vi "How to Calculate and Display Roots.vi"() -> ()   [LabVIEW 2020]
panel:
  out "Less Than 0":bool
  out "Greater than 0":bool
  out "D":dbl
  in  "C":dbl
  in  "B":dbl
  in  "A":dbl
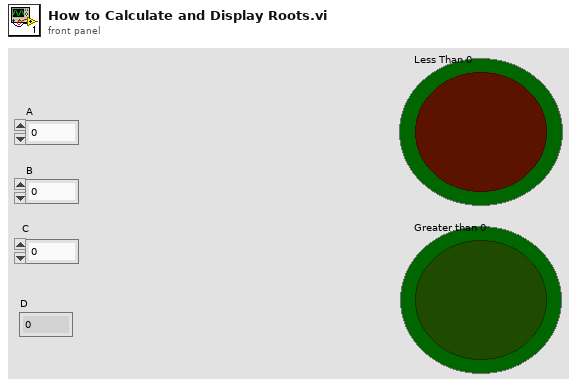
[diagram p1: front panel]
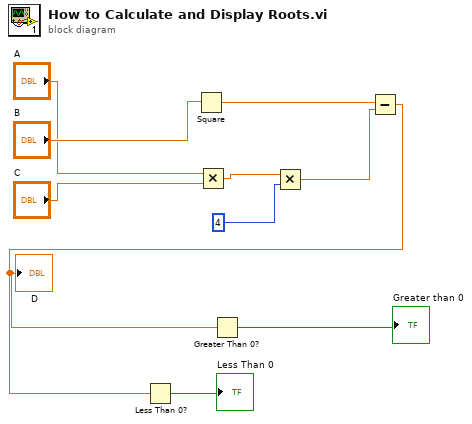
[diagram p0: block diagram]
diagram:
  n1 = Square(x="B") -> (x^2=w5:dbl)
  n2 = Multiply(x="A", y="C") -> (x*y=w7:dbl)
  n3 = Multiply(x=w7, y=4) -> (x*y=w4:dbl)
  n4 = Subtract(x=w5, y=w4) -> (x-y=w2:dbl)
  "D" <- w2
  n5 = Less Than 0?(x=w2) -> (x < 0?=→"Less Than 0":bool)
  n6 = Greater Than 0?(x=w2) -> (x > 0?=→"Greater than 0":bool)
